vi "DeviceSearch.vi"(8 "Error In":errorcluster caption="error in (no error)") -> (0 "Error Out":errorcluster, 2 "Devices":string[][](array[string]))   [LabVIEW 2023]
doc: "Searches through all connected VI devices and returns a string array of their names."
uses:
  <vilib>/nisyscfg/Close (System).vi
  <vilib>/nisyscfg/nisyscfg.lvlib
  <resource>/objmgr/nisysapi.rc
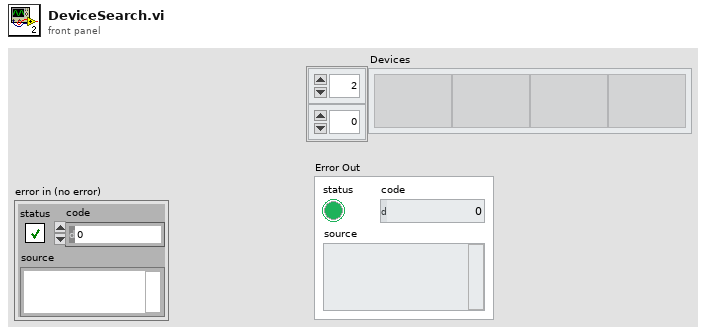
[diagram p1: front panel]
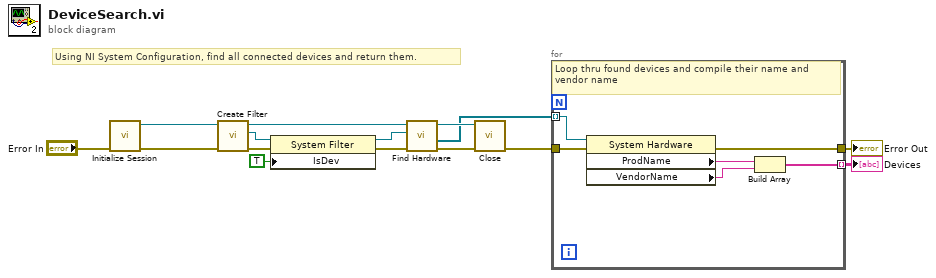
[diagram p0: block diagram]
diagram:
  # "Using NI System Configuration, find all connected devices and return them."
  n1 = call <vilib>:"Initialize Session.vi"("error in (no error)"="Error In") -> ("error out"=w11:errorcluster, "Session out"=w12:refnum<k21>)  [unwired: 9 in]
  n2 = call <vilib>:"Create Filter.vi"("error in (no error)"=w11, "Session in"=w12) -> ("error out"=w14:errorcluster, "Filter out"=w13:refnum<k20>, "Session out"=w7:refnum<k21>)  [unwired: 7 in]
  n3 = property class="System Filter"(reference=w13, error in=w14, "IsDev"=TRUE ("Is Device")) -> (reference out=w9:refnum<k20>, error out=w8:errorcluster)
  n4 = call <vilib>:"Find Hardware.vi"("error in (no error)"=w8, "Filter in"=w9, "Session in"=w7) -> ("error out"=w5:errorcluster, "Resources out"=w4:refnum<k20>[], "Session out"=w6:refnum<k21>)  [unwired: 5 in, 1 out]
  n5 = call-poly <vilib>:"Close.vi"("error in (no error)"=w5, "Session in"=w6) -> ("error out"=w3:errorcluster)  [unwired: 9 in]
  n6 = for {
    tunnel: w4 -> [w21] mode=indexing
    tunnel: w3 -> [w20]
    tunnel: [w17] -> w1 mode=indexing
    tunnel: [w16] -> w2
    # "Loop thru found devices and compile their name and vendor name"
    n7 = property class="System Hardware"(reference=w21, error in=w20) -> (error out=w16:errorcluster, "ProdName"=w19:string, "VendorName"=w18:string)  [unwired: 1 out]
    n8 = Build Array(w19, w18) -> (w17:string[])
  }
  "Error Out" <- w2
  "Devices" <- w1
